vi "Restore Defaults.vi"(8 "error in (no error)":errorcluster, 11 "Session Handle in":T1) -> (0 "error out":errorcluster, 3 "Session Handle out":T1)   [LabVIEW 2016, in "niRFUtil.lvlib" / "niRFUtil Session.lvclass"]
uses:
  niRFUtil Session.lvclass
  Includes/niRFUtil INC Session Handle.ctl
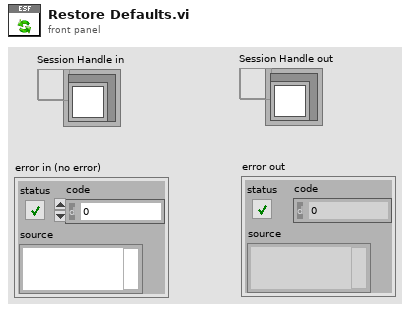
[diagram p1: front panel]
types:
  T1 = typedef "niRFUtil.lvlib/niRFUtil Session.lvclass/niRFUtil INC Session Handle.ctl" = refnum<data-value>
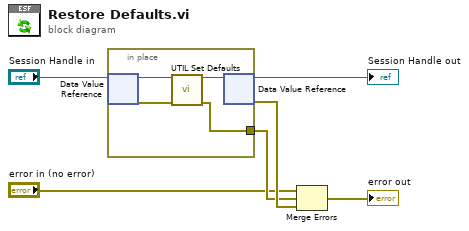
[diagram p0: block diagram]
diagram:
  n1 = in-place {
    in-place-border: [w7] -> w5
    n2 = in-place-dvr #1("Session Handle in") -> (w10:refnum<class "niRFUtil Session.lvclass">, w9:errorcluster)
    n3 = call-dynamic "UTIL Set Defaults.vi"("OBJ - Session in"=w10, "error in"=w9) -> ("OBJ - Session out"=w8:refnum<class "niRFUtil Session.lvclass">, "error out"=w7:errorcluster)  [unwired: 12 in]
    n4 = in-place-dvr #1(w8) -> (→"Session Handle out":T1, w6:errorcluster)
  }
  n5 = Merge Errors("error in (no error)", w5, w6) -> (→"error out":errorcluster)
